vi "ddot - Dot Product (DBL).vi"(5 "yInc":i32=1, 7 "xInc":i32=1, 10 "y":dbl[](array[numeric]), 11 "x":dbl[](array[numeric])) -> (0 "error":i32, 3 "ddot":dbl)   [LabVIEW 2017, in "NI_AALBLAS.lvlib"]
doc: "Calculates the dot product of two real vectors."
uses:
  NI_AALBLAS.lvlib
  Fucntion.ctl
  BLAS1 Utility(DBL).vi
panel:
  # "ddot=x'*y"
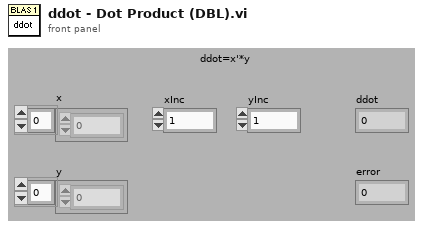
[diagram p1: front panel]
types:
  T1 = typedef "NI_AALBLAS.lvlib/Fucntion.ctl" = u16
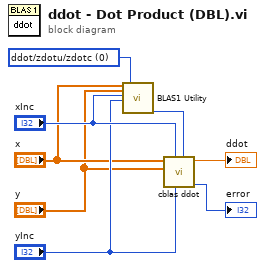
[diagram p0: block diagram]
diagram:
  w2 = T1 0 items=["ddot/zdotu/zdotc", "daxpy/zaxpy", "dnrm2/dznrm2", "dasum/dzasum", "dcopy/zcopy", "dswap/zswap", "drotm", "drot/zdrot", "idamax/izamax", "idamin/izamin", "dgemv/zgemv", "dsymv/zhemv", "dtrmv/ztrmv", "dsyr/zher", "dsyr2/zher2", "dger/zgeru/zgerc", "dtrsv/ztrsv", "dgemm/zgemm", "dsymm/zsymm/zhemm", "dtrmm/ztrmm", "dsyrk/zsyrk/zherk", "dsyr2k/zsyr2k/zher2k", "dtrsm/ztrsm"] ("function")
  n1 = call-poly "BLAS1 Utility.vi"("x"="x", "y"="y", "xInc"="xInc", "yInc"="yInc", "function"=w2) -> ("n"=w1:i32)  [unwired: 14 out]
  n2 = call "cblas ddot.vi"("n"=w1, "incy"="yInc", "incx"="xInc", "y"="y", "x"="x") -> ("error"=→"error":i32, "ddot"=→"ddot":dbl)  [unwired: 5 out]
